vi "Stop Core.vi"(10 "final error code":i32, 11 "TCP_Client in":refnum<class "TCP_Client.lvclass">) -> (3 "TCP_Client out":refnum<class "TCP_Client.lvclass">)   [LabVIEW 2023, in "TCP_Client.lvlib" / "TCP_Client.lvclass"]
doc: "(<B>Filename</B>: Actor Framework.lvlib:Actor.lvclass:Stop Core.vi)\n\nDefines what the actor does before it stops. Use the <B>final error code</B> input to determine whether the actor shut down in response to an error.\n\nBy default, this method passes the Stop message along to all auto-stop nested actors. A descendant class may override this method to define additional behavior, such as shutting down any processes the actor initiated in its override of the Actor Core method."
uses:
  TCP_Client.lvclass
  TCP_Client.lvclass/TCP_Client.ctl
  <vilib>/ActorFramework/Actor/Actor.lvclass
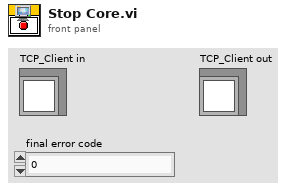
[diagram p1: front panel]
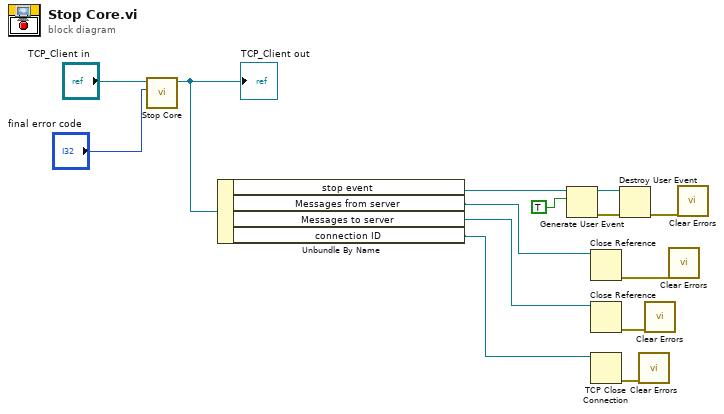
[diagram p0: block diagram]
diagram:
  n1 = call-parent "Stop Core.vi"("final error code"="final error code", "Actor in"="TCP_Client in") -> ("Actor out"=w12:refnum<class "TCP_Client.lvclass">)  [unwired: 9 in]
  "TCP_Client out" <- w12
  n2 = Unbundle By Name(w12) -> ("stop event"=w11:refnum<user-event>, "Messages from server"=w7:refnum<vi>, "Messages to server"=w6:refnum<vi>, "connection ID"=w5:refnum<k5>)
  n3 = Generate User Event(user event=w11, event data cluster=TRUE ("event data")) -> (user event out=w8:refnum<user-event>, error out=w9:errorcluster)  [unwired: 2 in]
  n4 = Close Reference(reference=w7) -> (error out=w2:errorcluster)  [unwired: 1 in]
  n5 = Close Reference(reference=w6) -> (error out=w1:errorcluster)  [unwired: 1 in]
  n6 = TCP Close Connection(connection ID=w5) -> (error out=w4:errorcluster)  [unwired: 2 in, 1 out]
  n7 = Destroy User Event(user event=w8, error in=w9) -> (error out=w3:errorcluster)
  n8 = call <vilib>:"Clear Errors.vi"("error in (no error)"=w4) -> ()  [unwired: 5 in, 2 out]
  n9 = call <vilib>:"Clear Errors.vi"("error in (no error)"=w1) -> ()  [unwired: 5 in, 2 out]
  n10 = call <vilib>:"Clear Errors.vi"("error in (no error)"=w2) -> ()  [unwired: 5 in, 2 out]
  n11 = call <vilib>:"Clear Errors.vi"("error in (no error)"=w3) -> ()  [unwired: 5 in, 2 out]
